vi "SetNavigationLevel.vi"(8 "ErrorIn":errorcluster caption="Error In", 9 "NavigationName":string, 10 "Authorization":refnum<class "IAuthorization.lvclass">, 11 "ObjectIn":refnum<class "ButtonCollection.lvclass"> caption="Object In") -> (0 "ErrorOut":errorcluster caption="Error Out", 3 "ObjectOut":refnum<class "ButtonCollection.lvclass"> caption="Object Out")   [LabVIEW 2021, in "ButtonCollection.lvclass"]
uses:
  ButtonCollection.lvclass
  .Externals/Interface_TAF_IAuthorization/IAuthorization/IAuthorization.lvclass
  ButtonCollection.lvclass/ButtonCollection.ctl
  747b0e3d-e3dc-4904-9170-8489d60c6556.vi
  <vilib>/TriekselSoft/TracerLibrary/TracerLibrary/Tracer/protected/SendMessage.vi
  <vilib>/TriekselSoft/TracerLibrary/TracerLibrary/Tracer/protected/Timestamp.vi
  747b0e3d-e3dc-4904-9170-8489d60c6556.vi/f75db090-0877-4668-94fb-75c2140b1617.vi
  <vilib>/TriekselSoft/TracerLibrary/TracerLibrary/Tracer/Tracer_Level-Debug.vi
  <vilib>/JDP Science/JSONtext/Variant to JSON Text.vi
  <vilib>/TriekselSoft/TracerLibrary/TracerLibrary/Tracer/protected/Tracer_ClassAttributes.vi
  <vilib>/JDP Science/JSONtext/LVClass Serializer/JSONtext LVClass Serializer.lvclass
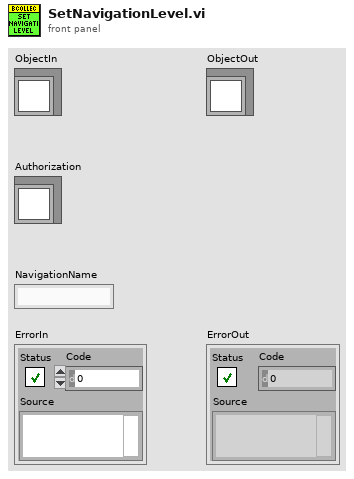
[diagram p1: front panel]
types:
  T1 = enum8{"Enabled", "Disabled", "Disabled and Grayed Out"}
  T2 = cluster{"Caption":string, "Eval":cluster{string, "Expression":string, "NotFoundLabels":string[], "ResultPerLabel":string[]}}
  T3 = typedef "ButtonCollection.lvclass/ButtonDefinition.ctl" = cluster{"ThisNavigationName":string, "ButtonLabel":string, "Caption":string, "Tooltip":string, "EnabledExpression":string, "Actions":cluster{"ActionType":string, "TargetObject":string, "Parameter":string, "WaitUntilDone":bool}[], "NextNavigationName":string}
  T4 = cluster{string, "Expression":string, "NotFoundLabels":string[], "ResultPerLabel":string[]}
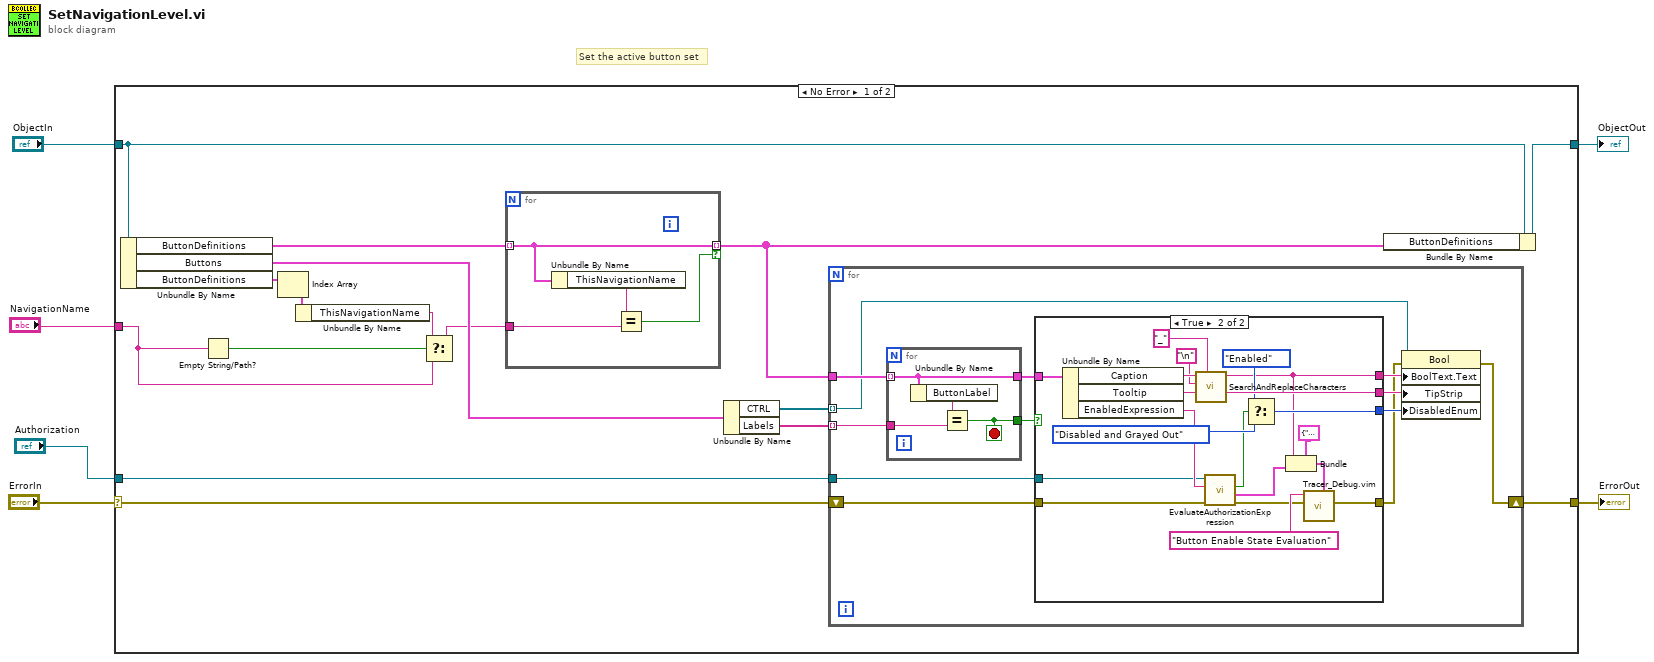
[diagram p0: block diagram]
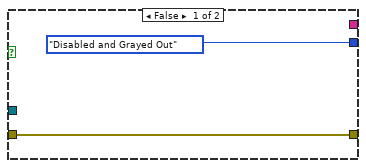
[diagram p2: hidden frame]
diagram:
  # "Set the active button set"
  n1 = case shown="No Error" "ErrorIn" {
    selector: "ErrorIn" -> [w15 w65]
    tunnel: [w14 w65] -> w5
    tunnel: [w20 w64] -> w3
    tunnel: "ObjectIn" -> [w22 w64]
    tunnel: "NavigationName" -> [w7 _]
    tunnel: "Authorization" -> [w13 _]
    frame No Error {
      n2 = Unbundle By Name(w22) -> ("ButtonDefinitions"=w21:T3[], "Buttons"=w19:cluster{"Labels":string[], "CTRL":refnum<vi>[]}, "ButtonDefinitions"=w12:T3[])
      n3 = Empty String/Path?(string/path=w7) -> (empty?=w10:bool)
      n4 = Index Array(array=w12) -> (element=w11:T3)  [unwired: 1 in]
      n5 = Unbundle By Name(w11) -> ("ThisNavigationName"=w9:string)
      n6 = Select(t=w9, s=w10, f=w7) -> (s? t:f=w8:string)
      n7 = for {
        tunnel: w21 -> [w24] mode=indexing
        tunnel: w8 -> [w25]
        tunnel: [w24] -> w17 mode=indexing if=w23
        n8 = Unbundle By Name(w24) -> ("ThisNavigationName"=w26:string)
        n9 = Equal?(x=w26, y=w25) -> (x = y?=w23:bool)
      }
      n10 = Unbundle By Name(w19) -> ("CTRL"=w16:refnum<vi>[], "Labels"=w18:string[])
      n11 = for {
        tunnel: w18 -> [w37] mode=indexing
        tunnel: w17 -> [w38]
        tunnel: w16 -> [w31] mode=indexing
        shift-right: [w30] -> w14
        shift-left: w15 -> [w29]
        tunnel: w13 -> [w27]
        n12 = for {
          tunnel: w38 -> [w60] mode=indexing
          tunnel: w37 -> [w63]
          tunnel: [w61] -> w36
          tunnel: [w60] -> w35
          stop <- w61 stop-if-true
          n13 = Unbundle By Name(w60) -> ("ButtonLabel"=w62:string)
          n14 = Equal?(x=w62, y=w63) -> (x = y?=w61:bool)
        }
        n15 = case shown="True" w36 {
          tunnel: w35 -> [_ w59]
          tunnel: [_ w46] -> w34
          tunnel: [_ w57] -> w33
          tunnel: [T1."Disabled and Grayed Out" ("Disabled") w56] -> w32
          tunnel: [w39 w47] -> w28
          tunnel: w29 -> [w39 w53]
          tunnel: w27 -> [_ w41]
          frame False {
          }
          frame True {
            n16 = Unbundle By Name(w59) -> ("Caption"=w58:string, "Tooltip"=w57:string, "EnabledExpression"=w52:string)
            n17 = call "SearchAndReplaceCharacters.vi"("CharactersToSearch"="_", "CharacterToReplace"="\n", "string in"=w58) -> ("result string"=w46:string)  [unwired: 8 in]
            n18 = call-dynamic "EvaluateAuthorizationExpression.vi"("Error In"=w53, "Expression"=w52, "reference in"=w41) -> ("Error Out"=w48:errorcluster, "Result"=w45:T4, "Pass"=w51:bool)  [unwired: 5 in, 1 out]
            n19 = Select(t=T1."Enabled" ("Disabled"), s=w51, f=T1."Disabled and Grayed Out" ("Disabled")) -> (s? t:f=w56:T1)
            n20 = Bundle(cluster=T2 {"Caption"="", "Eval"={"", "Expression"="", "NotFoundLabels"=[], "ResultPerLabel"=[]}}, "Caption"=w46, "Eval"=w45) -> (w44:T2)
            n21 = call "Tracer_Debug.vim"("Data"=w44, "error in (no error)"=w48, "Text"="Button Enable State Evaluation") -> ("error out"=w47:errorcluster)  [unwired: 8 in]
          }
        }
        n22 = property class="Bool"(reference=w31, error in=w28, "BoolText.Text"=w34, "TipStrip"=w33, "DisabledEnum"=w32) -> (error out=w30:errorcluster)  [unwired: 1 out]
      }
      n23 = Bundle By Name(cluster=w22, "ButtonDefinitions"=w17) -> (w20:refnum<class "ButtonCollection.lvclass">)
    }
    frame Error {
    }
  }
  "ErrorOut" <- w5
  "ObjectOut" <- w3
